vi "test_TCP_1_RT.vi"() -> ()   [LabVIEW 2014]
panel:
  out "error out 2":errorcluster
  out "error out":errorcluster
  in  "stop":bool
  out "string":string
  out "type_cast":string
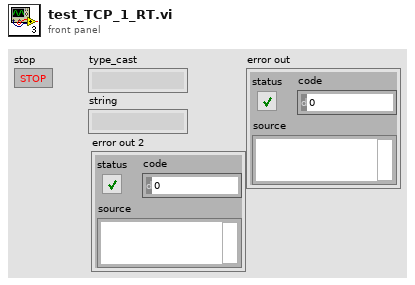
[diagram p1: front panel]
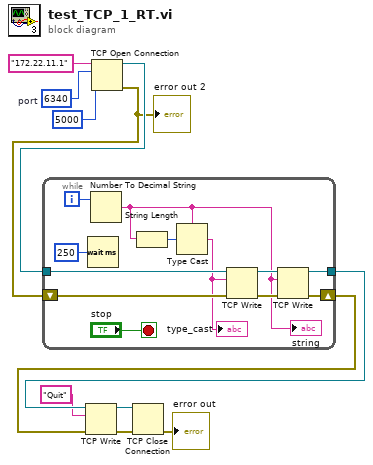
[diagram p0: block diagram]
diagram:
  w11 = u16 6340  # port
  n1 = TCP Open Connection(address="172.22.11.1", remote port or service name=w11, timeout ms (60000)=5000) -> (connection ID=w9:refnum<k5>, error out=w8:errorcluster)  [unwired: 2 in]
  "error out 2" <- w8
  n2 = while {
    tunnel: w9 -> [w20]
    shift-right: [w16] -> w6
    shift-left: w8 -> [w19]
    tunnel: [w14] -> w5
    i -> [w22]
    stop <- "stop" stop-if-true
    n3 = Wait (ms)(milliseconds to wait=u32 250) -> ()  [unwired: 1 out]
    n4 = Number To Decimal String(number=w22) -> (decimal integer string=w13:string)  [unwired: 1 in]
    "string" <- w13
    n5 = String Length(string=w13) -> (length=w21:i32)
    n6 = Type Cast(type=w13, x=w21) -> (*(type *) &x=w18:string)
    "type_cast" <- w18
    n7 = TCP Write(connection ID=w20, data in=w18, error in (no error)=w19) -> (connection ID out=w15:refnum<k5>, error out=w17:errorcluster)  [unwired: 2 out]
    n8 = TCP Write(connection ID=w15, data in=w13, error in (no error)=w17) -> (connection ID out=w14:refnum<k5>, error out=w16:errorcluster)  [unwired: 2 out]
  }
  n9 = TCP Write(connection ID=w5, data in="Quit", error in (no error)=w6) -> (connection ID out=w4:refnum<k5>, error out=w7:errorcluster)  [unwired: 2 out]
  n10 = TCP Close Connection(connection ID=w4, error in (no error)=w7) -> (error out=→"error out":errorcluster)  [unwired: 1 in, 1 out]
